vi "Simulation Lab -Array - B220061.vi"() -> ()   [LabVIEW 2020]
panel:
  out "Array":dbl[](array[numeric])
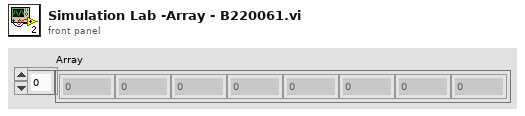
[diagram p1: front panel]
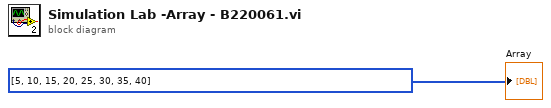
[diagram p0: block diagram]
diagram:
  "Array" <- i32[] [5, 10, 15, 20, 25, 30, 35, 40]
